vi "质控关于.vi"(11 "Slave ID":T1) -> ()   [LabVIEW 2016, in "质控单元V2.lvlib"]
panel:
  in  "关闭":bool
  out "固件状态：":string
  out "固件信息：":string
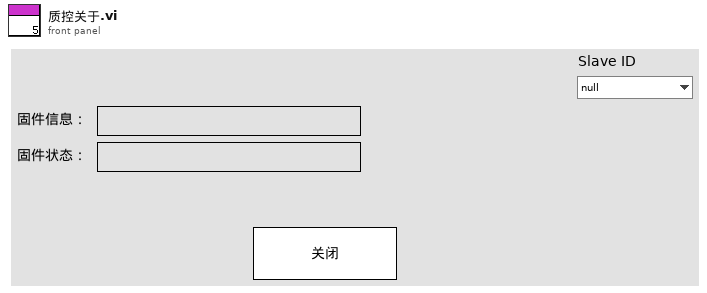
[diagram p1: front panel]
types:
  T1 = typedef "质控单元V2.lvlib/质控slave id.ctl" = enum16{"null", "氨氮", "总磷", "总氮", "CODMn", "CODCr"}
  T2 = typedef "质控单元V2.lvlib/固件状态.ctl" = u16
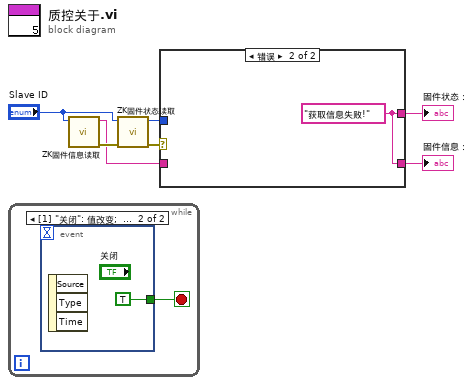
[diagram p0: block diagram]
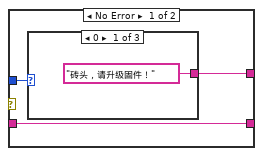
[diagram p2: hidden frame]
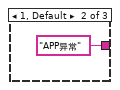
[diagram p3: hidden frame]
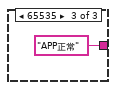
[diagram p4: hidden frame]
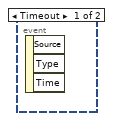
[diagram p5: hidden frame]
diagram:
  n1 = while {
    stop <- w8 stop-if-true
    n2 = event shown="[1] \"关闭\": 值改变;  前面板关闭" {
      selector: _ -> [_ _]
      dyn-events: _ -> [_ _]
      timeout: _ -> [_ _]
      tunnel: [_ TRUE] -> w8
      event Timeout {
        n3 = event-data() -> ()  [unwired: 1 in, 3 out]
      }
      event "关闭": Value Change; Panel Close {
        n4 = event-data() -> ()  [unwired: 1 in, 3 out]
      }
    }
  }
  n5 = call "ZK固件信息读取.vi"("Slave ID"="Slave ID") -> ("error out"=w6:errorcluster, "固件信息"=w1:string)  [unwired: 9 in]
  n6 = call "ZK固件状态读取.vi"("error in (no error)"=w6, "Slave ID"="Slave ID") -> ("error out"=w3:errorcluster, "固件状态"=w5:T2)  [unwired: 8 in]
  n7 = case shown="错误" w3 {
    tunnel: w5 -> [w12 _]
    tunnel: [w11 w16] -> w4
    tunnel: [w10 w16] -> w2
    tunnel: w1 -> [w10 _]
    frame No Error {
      n8 = case shown="0" w12 {
        tunnel: ["砖头，请升级固件！" ("固件状态：") "APP异常" ("固件状态：") "APP正常" ("固件状态：")] -> w11
        frame 0 {
        }
        frame 1, Default {
        }
        frame 65535 {
        }
      }
    }
    frame Error {
      w16 = "获取信息失败!" ("固件信息")
    }
  }
  "固件信息：" <- w2
  "固件状态：" <- w4
